vi "RFIDGetLastTag.vi"(8 "error in (no error)":errorcluster, 11 "Device In":u64) -> (0 "error out":errorcluster, 1 "Protocol":i32(ring) items=["PROTOCOL_EM4100"=1, "PROTOCOL_ISO11785_FDX_B"=2, "PROTOCOL_PHIDGETS"=3], 2 "Tag String":string, 3 "Device Out":u64)   [LabVIEW 2012, in "Phidget RFID.lvlib"]
doc: "${GetLastTag:Header}"
uses:
  <instrlib>/Phidgets/Phidget RFID/Phidget RFID.lvlib
  <instrlib>/Phidgets/Phidget Common/Phidget Common.lvlib
  phidget22.dll
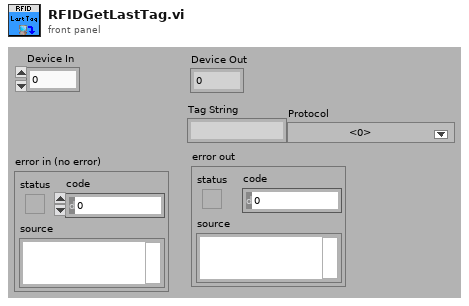
[diagram p1: front panel]
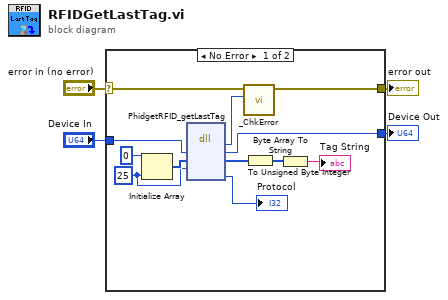
[diagram p0: block diagram]
diagram:
  n1 = case shown="No Error" "error in (no error)" {
    selector: "error in (no error)" -> [w14 w18]
    tunnel: [w13 w18] -> w3
    tunnel: "Device In" -> [w16 w17]
    tunnel: [w15 w17] -> w1
    frame No Error {
      w9 = 25 ("dimension size")
      n2 = Initialize Array(u8 0 ("element"), w9) -> (w11:u8[])
      n3 = dll-call lib="phidget22.*" fn="PhidgetRFID_getLastTag"("phid"=w16, "Tag"=w11, "tagStrLen"=w9) -> ("return type"=w12:i32, "phid"=w15:u64, "Tag"=w8:u8[], "protocol"=→"Protocol":i32)  [unwired: 5 in, 2 out]
      n4 = call <instrlib>:"_ChkError.vi"("Return Code"=w12, "error in (no error)"=w14) -> ("error out"=w13:errorcluster)  [unwired: 9 in]
      n5 = To Unsigned Byte Integer(number=w8) -> (unsigned 8bit integer=w6:u8[])
      n6 = Byte Array To String(unsigned byte array=w6) -> (string=→"Tag String":string)
    }
    frame Error {
    }
  }
  "error out" <- w3
  "Device Out" <- w1
